vi "KickForce.vi"(0 "KickToSkill in":refnum<class "KickToSkill.lvclass">, 1 "Enviroment":T1, 2 "Ball":refnum<class "Ball.lvclass">, 3 "weakForce":dbl format="%#_13g", 5 "force++":dbl, 9 "Distance to target":dbl, 11 "error in (no error)":errorcluster, 12 "kickForce":dbl, 13 "weakKick?":bool=TRUE, 14 "pass?":bool=TRUE) -> (4 "KickToSkill out":refnum<class "KickToSkill.lvclass">, 10 "Force":dbl, 15 "error out":errorcluster)   [LabVIEW 2020, in "KickToSkill.lvclass"]
uses:
  KickToSkill.lvclass
  Game_class/Game.lvclass
  Controls/Enviroment.ctl
  Ball_class/Ball.lvclass
  Field_class/Field.lvclass
panel:
  in  "Field":refnum<class "Field.lvclass">
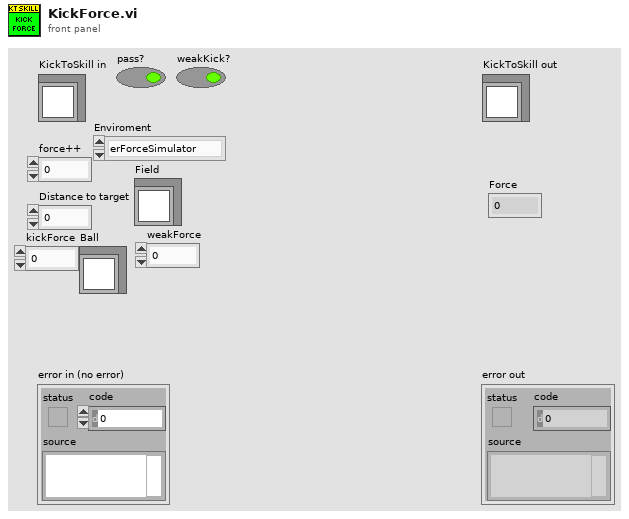
[diagram p1: front panel]
types:
  T1 = typedef "Enviroment.ctl" = enum16{"erForceSimulator", "grSim", "realGame"}
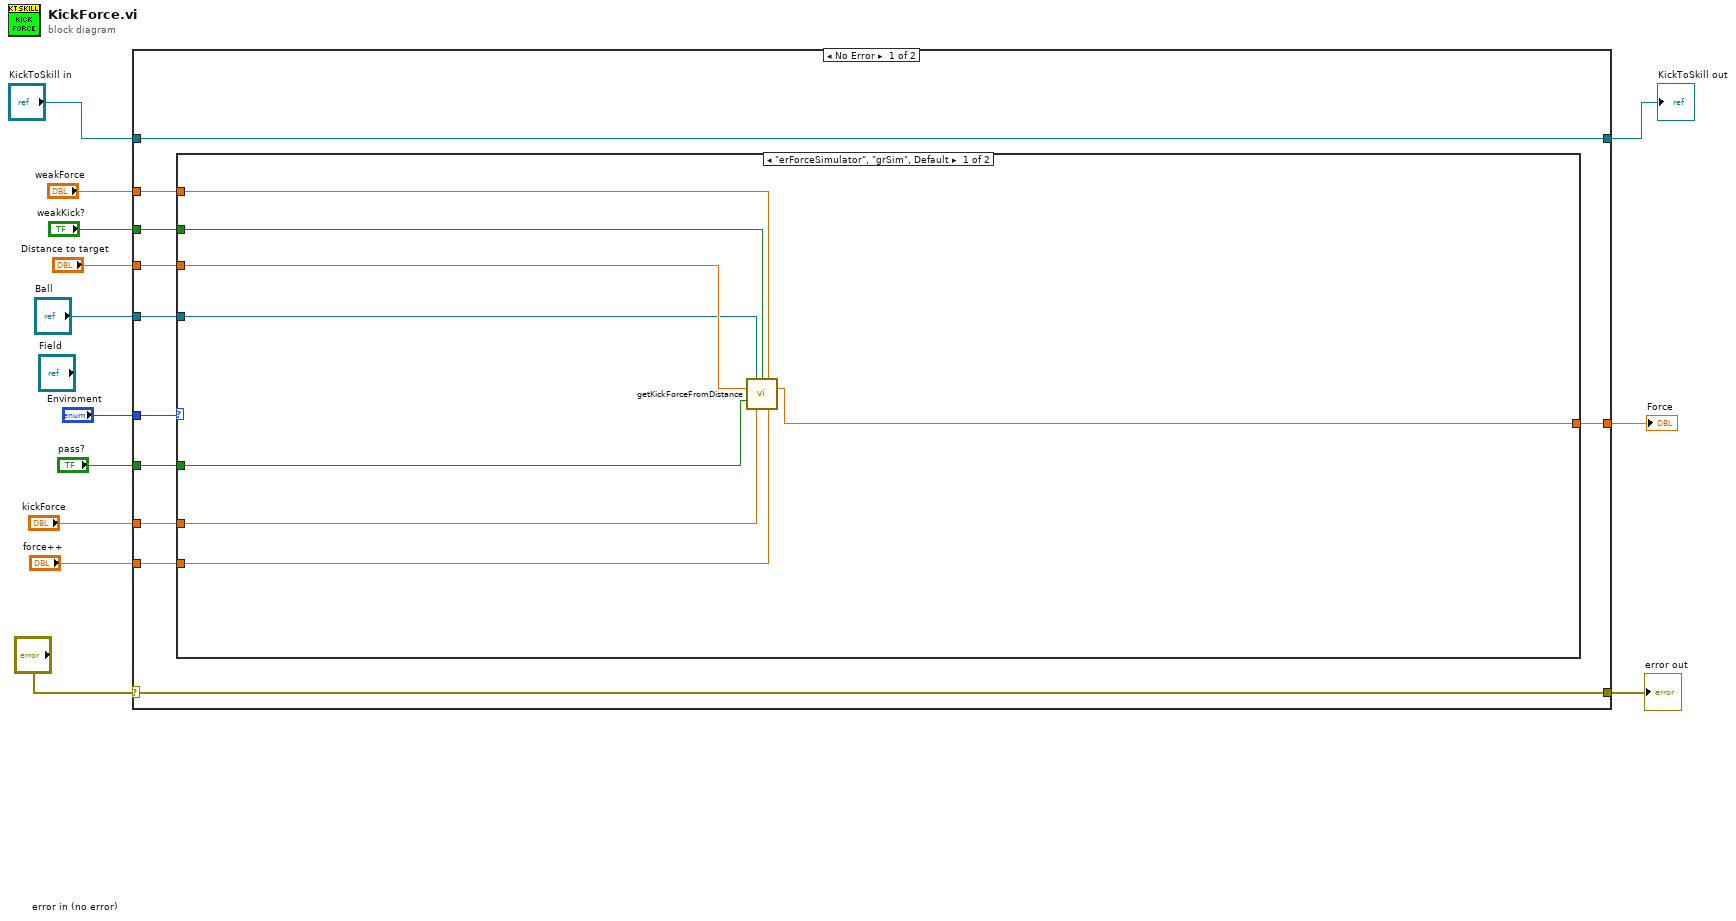
[diagram p0: block diagram]
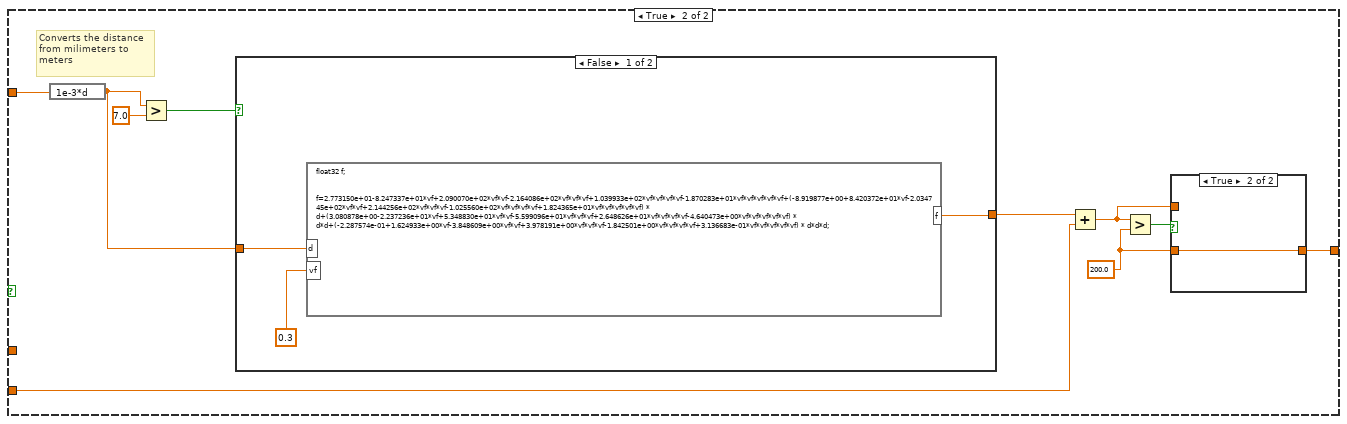
[diagram p3: hidden frame]
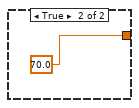
[diagram p5: hidden frame]
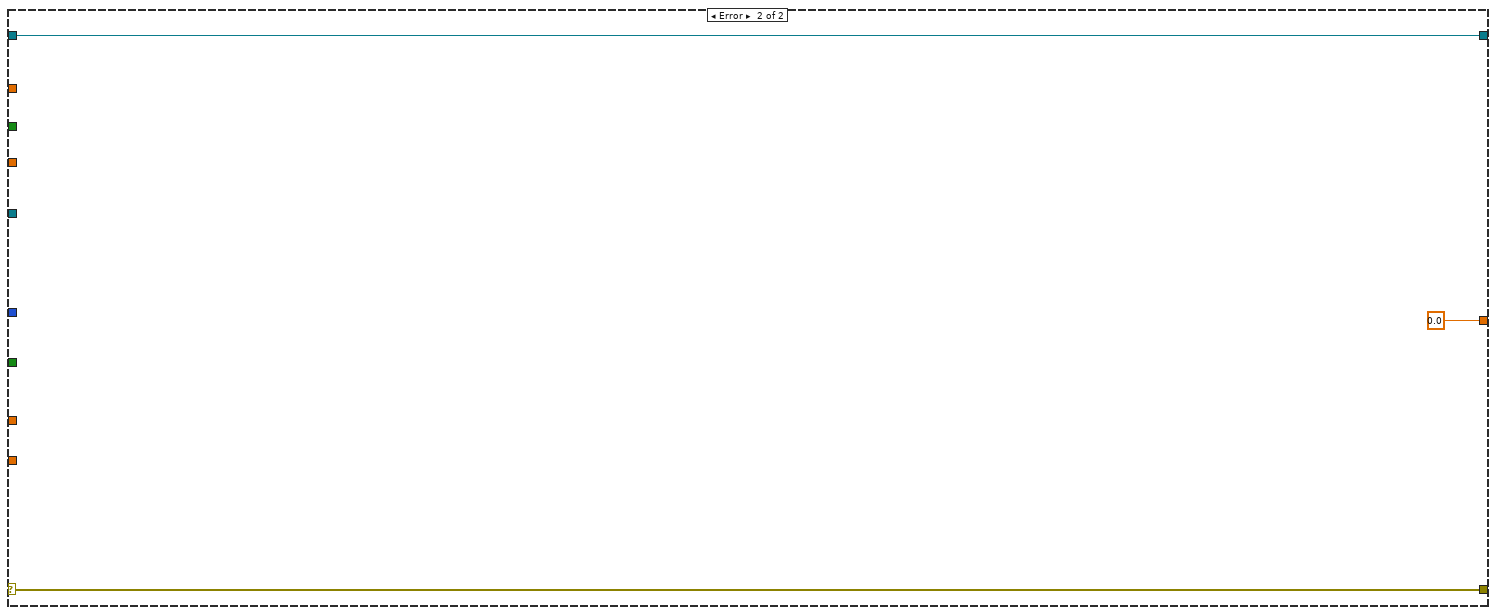
[diagram p6: hidden frame]
diagram:
  n1 = case shown="No Error" "error in (no error)" {
    selector: "error in (no error)" -> [w23 w57]
    tunnel: [w23 w57] -> w12
    tunnel: [w24 w56] -> w10
    tunnel: "KickToSkill in" -> [w24 w56]
    tunnel: "Distance to target" -> [w22 _]
    tunnel: [w21 0.0 ("y")] -> w8
    tunnel: "Enviroment" -> [w20 _]
    tunnel: "force++" -> [w19 _]
    tunnel: "pass?" -> [w18 _]
    tunnel: "kickForce" -> [w17 _]
    tunnel: "Ball" -> [w16 _]
    tunnel: "weakForce" -> [w15 _]
    tunnel: "weakKick?" -> [w14 _]
    frame No Error {
      n2 = case shown="\"erForceSimulator\", \"grSim\", Default" w20 {
        tunnel: w22 -> [w30 w37]
        tunnel: [w31 w36] -> w21
        tunnel: w19 -> [w28 w35]
        tunnel: w18 -> [w32 w34]
        tunnel: w17 -> [w29 w33]
        tunnel: w16 -> [w27 _]
        tunnel: w15 -> [w26 _]
        tunnel: w14 -> [w25 _]
        frame "erForceSimulator", "grSim", Default {
          n3 = call "getKickForceFromDistance.vi"("Ball"=w27, "weakKick?"=w25, "weakKickForce"=w26, "distance"=w30, "pass?"=w32, "KickForce"=w29, "multiplicativeFactorToPassForce"=w28) -> ("kickForce"=w31:dbl)  [unwired: 6 in, 2 out]
        }
        frame "realGame" {
          n4 = case shown="False" w34 {
            tunnel: w37 -> [_ w48]
            tunnel: [w38 w42] -> w36
            tunnel: w35 -> [_ w39]
            tunnel: w33 -> [w38 _]
            frame False {
            }
            frame True {
              w41 = 200.0 ("y")
              # "Converts the distance\nfrom milimeters to \nmeters"
              n5 = expression code="1e-3*d"(w48) -> (w45:dbl)
              n6 = Greater?(x=w45, y=7.0) -> (0:w47:bool)
              n7 = case shown="False" w47 {
                tunnel: [w52 70.0] -> w44
                tunnel: w45 -> [w51 _]
                frame False {
                  n8 = formula code="float32 f;\n\n\nf=2.773150e+01-8.247337e+01*vf+2.090070e+02*vf*vf-2.164086e+02*vf*vf*vf+1.039933e+02*vf*vf*vf*vf-1.870283e+01*vf*vf*vf*vf*vf+(-8.919877e+00+8.420372e+01*vf-2.034745e+02*vf*vf+2.144256e+02*vf*vf*vf-1.025560e+02*vf*vf*vf*vf+1.824365e+01*vf*vf*vf*vf*vf) * d+(3.080878e+00-2.237236e+01*vf+5.348830e+01*vf*vf-5.599096e+01*vf*vf*vf+2.648626e+01*vf*vf*vf*vf-4.640473e+00*vf*vf*vf*vf*vf) * d*d+(-2.287574e-01+1.624933e+00*vf-3.848609e+00*vf*vf+3.978191e+00*vf*vf*vf-1.842501e+00*vf*vf*vf*vf+3.136683e-01*vf*vf*vf*vf*vf) * d*d*d;"("d"=w51, "vf"=0.3 ("input variable")) -> ("f"=w52:sgl)
                }
                frame True {
                }
              }
              n9 = Add(x=w44, y=w39) -> (x+y=w40:dbl)
              n10 = Greater?(x=w40, y=w41) -> (0:w43:bool)
              n11 = case shown="True" w43 {
                tunnel: [w49 w50] -> w42
                tunnel: w41 -> [_ w50]
                tunnel: w40 -> [w49 _]
                frame False {
                }
                frame True {
                }
              }
            }
          }
        }
      }
    }
    frame Error {
    }
  }
  "error out" <- w12
  "KickToSkill out" <- w10
  "Force" <- w8
